vi "Special Write.vi"(8 "error in (no error)":errorcluster, 9 "Delay (0 ms)":u32 max=3000, 10 "Input String":string, 11 "VISA resource name":refnum<visa-resource-name>) -> (0 "error out":errorcluster, 3 "VISA resource name out":refnum<visa-resource-name>)   [LabVIEW 2018, in "BK Precision 983X Series.lvlib"]
doc: "Performs a VISA write with a specified delay after the write operation."
uses:
  <instrlib>/BK Precision 983X Series/BK Precision 983X Series.lvlib
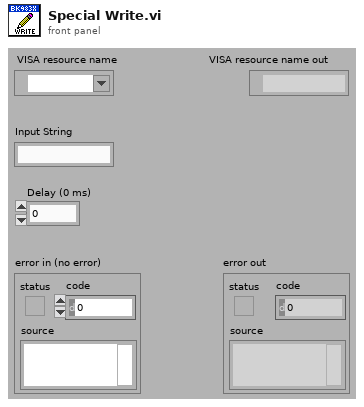
[diagram p1: front panel]
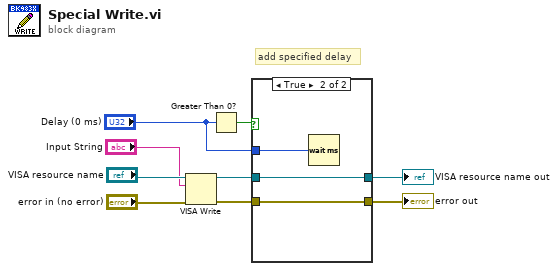
[diagram p0: block diagram]
diagram:
  # "add specified delay"
  n1 = VISA Write(VISA resource name="VISA resource name", write buffer="Input String", error in (no error)="error in (no error)") -> (VISA resource name out=w5:refnum<visa-resource-name>, error out=w4:errorcluster)  [unwired: 1 out]
  n2 = Greater Than 0?(x="Delay (0 ms)") -> (x > 0?=w2:bool)
  n3 = case shown="True" w2 {
    tunnel: [w11 w14] -> w6
    tunnel: w5 -> [w11 w14]
    tunnel: w4 -> [w10 w13]
    tunnel: [w10 w13] -> w3
    tunnel: "Delay (0 ms)" -> [_ w12]
    frame False {
    }
    frame True {
      n4 = Wait (ms)(milliseconds to wait=w12) -> ()  [unwired: 1 out]
    }
  }
  "error out" <- w3
  "VISA resource name out" <- w6
